vi "Robot Systems.vi"(11 "input cluster":T1) -> ()   [LabVIEW 2015]
uses:
  References/Refnums.vi
  Joystick/ControlsToCommands.ctl
panel:
  in  "Numeric":dbl
  out "YAxisLeft #2":dbl
  out "YAxisRight":dbl
  out "YAxisLeft":dbl
  out "XAxisLeft":dbl
  in  "Driving":u16(ring) items=["Manual", "Arcade", "Tank"]
  in  "Time Spinning before Index":dbl=5.0 caption="Delay Time (s)"
  in  "Time Indexing before Turning off Motors":dbl=3.0 caption="Delay Time (s)"
  in  "Motor Power":dbl min=-1.0 max=1.0 step=1.0
  in  "PWM 0":dbl min=-1.0 max=1.0
  in  "PWM 1":dbl min=-1.0 max=1.0
  in  "PWM 2":dbl min=-1.0 max=1.0
  in  "PWM 3":dbl min=-1.0 max=1.0
  in  "PWM 4":dbl min=-1.0 max=1.0
  in  "PWM 5":dbl min=-1.0 max=1.0
  in  "Apply Values":bool
  out "Boolean":bool
  in  "PWM 8":dbl min=-1.0 max=1.0 step=1.0
  # "THIS CANNOT BE ABORTED"
  # "MAYBE?"
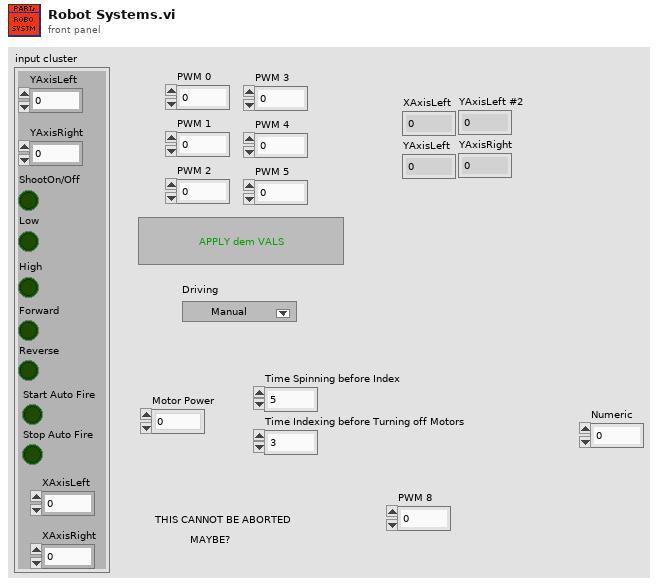
[diagram p1: front panel]
types:
  T1 = typedef "ControlsToCommands.ctl" = cluster{"YAxisLeft":dbl, "YAxisRight":dbl, "ShootOn/Off":bool, "Low":bool, "High":bool, "Forward":bool, "Reverse":bool, "Start Auto Fire":bool, "Stop Auto Fire":bool, "XAxisLeft":dbl, "XAxisRight":dbl}
  T2 = typedef "WPI_MotorControlDeviceRef.ctl" = cluster{"DeviceStatus":errorcluster, "Type":T3, "PWM":cluster{"PWM Channel":T4, "DeadBand":T5}, "CAN":cluster{"Device Number":u8, "Control Mode":T6, "Semaphore":T7, "Max Vout":dbl, "TalonSRX Control Mode":T8}, "Invert":bool}
  T3 = typedef "WPI_MotorControlType.ctl" = enum16{"PWM", "CAN", "CANTalonSRX"}
  T4 = typedef "FPGA_DIOPWMChannel.ctl" = enum8{"PWM 0", "PWM 1", "PWM 2", "PWM 3", "PWM 4", "PWM 5", "PWM 6", "PWM 7", "PWM 8", "PWM 9", "PWM MXP 0", "PWM MXP 1", "PWM MXP 2", "PWM MXP 3", "PWM MXP 4", "PWM MXP 5", "PWM MXP 6", "PWM MXP 7", "PWM MXP 8", "PWM MXP 9", "Invalid"}
  T5 = typedef "WPI_PWMDeadband.ctl" = cluster{"Name":string, "maxPositivePwm":i32, "minPositivePwm":i32, "centerPwm":i32, "maxNegativePwm":i32, "minNegativePwm":i32, "angularRange":u16}
  T6 = typedef "WPI_CANJaguar_ControlMode.ctl" = enum8{"Percent VBus", "Current", "Speed", "Position", "Voltage"}
  T7 = typedef "Semaphore RefNum" = refnum<k1>
  T8 = typedef "WPI_CANTalonSRX_APIControlMode.ctl" = enum8{"Percent VBus", "Speed", "Position", "Slave", "Unchanged / Invalid", "Voltage Compensation", "Current", "Motion Profile"}
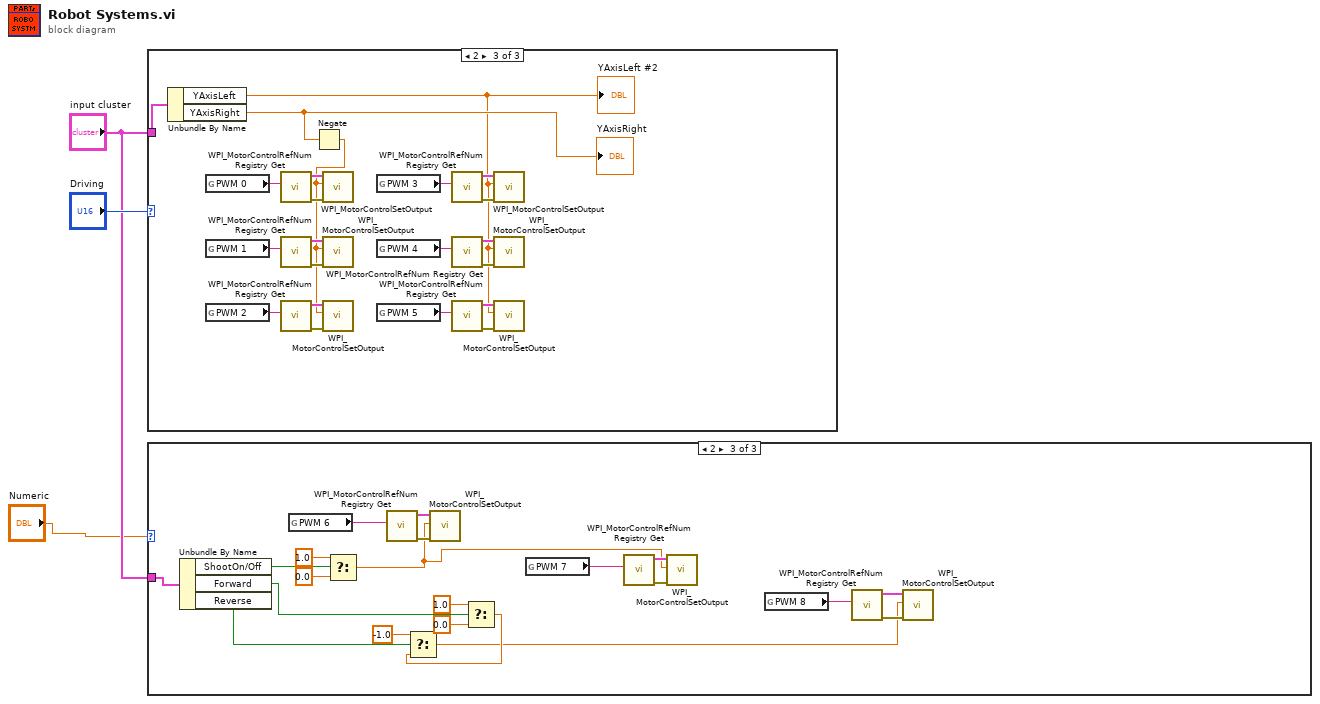
[diagram p0: block diagram]
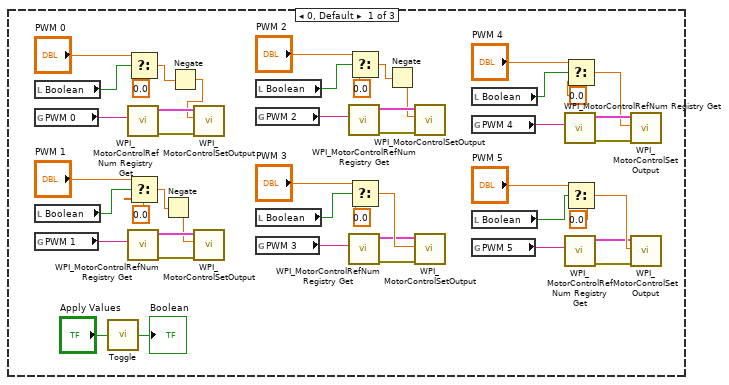
[diagram p2: hidden frame]
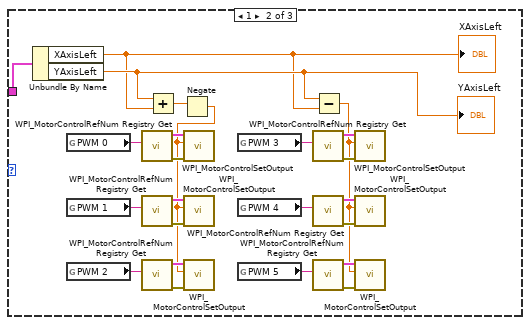
[diagram p3: hidden frame]
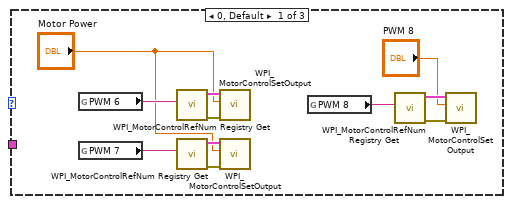
[diagram p4: hidden frame]
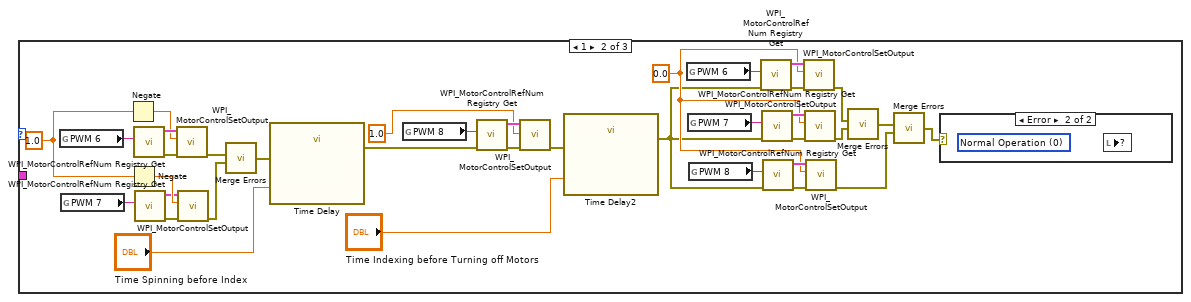
[diagram p5: hidden frame]
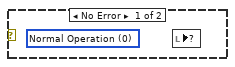
[diagram p6: hidden frame]
diagram:
  n1 = case shown="2" "Driving" {
    tunnel: "input cluster" -> [_ w74 w96]
    frame 0, Default {
      n2 = local read "Boolean"() -> (w34:bool)
      n3 = global read "Refnums.vi" "PWM 0"() -> (w23:string)
      n4 = local read "Boolean"() -> (w35:bool)
      n5 = global read "Refnums.vi" "PWM 1"() -> (w29:string)
      n6 = call "Toggle.vi"("Input"="Apply Values") -> ("Output"=→"Boolean":bool)  [unwired: 4 in]
      n7 = call <vilib>:"WPI_MotorControlRefNum Registry Get.vi"("refnum name"=w23) -> ("error out"=w25:errorcluster, "MotorControlDevRef"=w24:T2)  [unwired: 9 in]
      n8 = call <vilib>:"WPI_MotorControlRefNum Registry Get.vi"("refnum name"=w29) -> ("error out"=w31:errorcluster, "MotorControlDevRef"=w30:T2)  [unwired: 9 in]
      n9 = Select(t="PWM 0", s=w34, f=0.0) -> (s? t:f=w11:dbl)
      n10 = Select(t="PWM 1", s=w35, f=0.0) -> (s? t:f=w5:dbl)
      n11 = Negate(x=w5) -> (-x=w4:dbl)
      n12 = Negate(x=w11) -> (-x=w10:dbl)
      n13 = call <vilib>:"WPI_MotorControlSetOutput.vi"("error in (no error)"=w25, "Output"=w10, "MotorControlDevRef"=w24) -> ()  [unwired: 6 in, 3 out]
      n14 = call <vilib>:"WPI_MotorControlSetOutput.vi"("error in (no error)"=w31, "Output"=w4, "MotorControlDevRef"=w30) -> ()  [unwired: 6 in, 3 out]
      n15 = local read "Boolean"() -> (w37:bool)
      n16 = global read "Refnums.vi" "PWM 2"() -> (w28:string)
      n17 = local read "Boolean"() -> (w38:bool)
      n18 = global read "Refnums.vi" "PWM 3"() -> (w17:string)
      n19 = call <vilib>:"WPI_MotorControlRefNum Registry Get.vi"("refnum name"=w28) -> ("error out"=w26:errorcluster, "MotorControlDevRef"=w27:T2)  [unwired: 9 in]
      n20 = call <vilib>:"WPI_MotorControlRefNum Registry Get.vi"("refnum name"=w17) -> ("error out"=w19:errorcluster, "MotorControlDevRef"=w18:T2)  [unwired: 9 in]
      n21 = Select(t="PWM 2", s=w37, f=0.0) -> (s? t:f=w9:dbl)
      n22 = Select(t="PWM 3", s=w38, f=0.0) -> (s? t:f=w47:dbl)
      n23 = Negate(x=w9) -> (-x=w8:dbl)
      n24 = call <vilib>:"WPI_MotorControlSetOutput.vi"("error in (no error)"=w26, "Output"=w8, "MotorControlDevRef"=w27) -> ()  [unwired: 6 in, 3 out]
      n25 = call <vilib>:"WPI_MotorControlSetOutput.vi"("error in (no error)"=w19, "Output"=w47, "MotorControlDevRef"=w18) -> ()  [unwired: 6 in, 3 out]
      n26 = local read "Boolean"() -> (w41:bool)
      n27 = global read "Refnums.vi" "PWM 4"() -> (w16:string)
      n28 = local read "Boolean"() -> (w42:bool)
      n29 = global read "Refnums.vi" "PWM 5"() -> (w22:string)
      n30 = call <vilib>:"WPI_MotorControlRefNum Registry Get.vi"("refnum name"=w16) -> ("error out"=w14:errorcluster, "MotorControlDevRef"=w15:T2)  [unwired: 9 in]
      n31 = call <vilib>:"WPI_MotorControlRefNum Registry Get.vi"("refnum name"=w22) -> ("error out"=w20:errorcluster, "MotorControlDevRef"=w21:T2)  [unwired: 9 in]
      n32 = Select(t="PWM 4", s=w41, f=0.0) -> (s? t:f=w7:dbl)
      n33 = Select(t="PWM 5", s=w42, f=0.0) -> (s? t:f=w50:dbl)
      n34 = call <vilib>:"WPI_MotorControlSetOutput.vi"("error in (no error)"=w14, "Output"=w7, "MotorControlDevRef"=w15) -> ()  [unwired: 6 in, 3 out]
      n35 = call <vilib>:"WPI_MotorControlSetOutput.vi"("error in (no error)"=w20, "Output"=w50, "MotorControlDevRef"=w21) -> ()  [unwired: 6 in, 3 out]
    }
    frame 1 {
      n36 = Unbundle By Name(w74) -> ("XAxisLeft"=w54:dbl, "YAxisLeft"=w55:dbl)
      "XAxisLeft" <- w54
      "YAxisLeft" <- w55
      n37 = global read "Refnums.vi" "PWM 0"() -> (w70:string)
      n38 = global read "Refnums.vi" "PWM 1"() -> (w65:string)
      n39 = global read "Refnums.vi" "PWM 2"() -> (w58:string)
      n40 = call <vilib>:"WPI_MotorControlRefNum Registry Get.vi"("refnum name"=w70) -> ("error out"=w69:errorcluster, "MotorControlDevRef"=w68:T2)  [unwired: 9 in]
      n41 = call <vilib>:"WPI_MotorControlRefNum Registry Get.vi"("refnum name"=w65) -> ("error out"=w66:errorcluster, "MotorControlDevRef"=w67:T2)  [unwired: 9 in]
      n42 = call <vilib>:"WPI_MotorControlRefNum Registry Get.vi"("refnum name"=w58) -> ("error out"=w57:errorcluster, "MotorControlDevRef"=w56:T2)  [unwired: 9 in]
      n43 = Add(x=w55, y=w54) -> (x+y=w52:dbl)
      n44 = Negate(x=w52) -> (-x=w51:dbl)
      n45 = call <vilib>:"WPI_MotorControlSetOutput.vi"("error in (no error)"=w69, "Output"=w51, "MotorControlDevRef"=w68) -> ()  [unwired: 6 in, 3 out]
      n46 = call <vilib>:"WPI_MotorControlSetOutput.vi"("error in (no error)"=w66, "Output"=w51, "MotorControlDevRef"=w67) -> ()  [unwired: 6 in, 3 out]
      n47 = call <vilib>:"WPI_MotorControlSetOutput.vi"("error in (no error)"=w57, "Output"=w51, "MotorControlDevRef"=w56) -> ()  [unwired: 6 in, 3 out]
      n48 = global read "Refnums.vi" "PWM 3"() -> (w71:string)
      n49 = global read "Refnums.vi" "PWM 4"() -> (w64:string)
      n50 = global read "Refnums.vi" "PWM 5"() -> (w59:string)
      n51 = call <vilib>:"WPI_MotorControlRefNum Registry Get.vi"("refnum name"=w71) -> ("error out"=w73:errorcluster, "MotorControlDevRef"=w72:T2)  [unwired: 9 in]
      n52 = call <vilib>:"WPI_MotorControlRefNum Registry Get.vi"("refnum name"=w64) -> ("error out"=w62:errorcluster, "MotorControlDevRef"=w63:T2)  [unwired: 9 in]
      n53 = call <vilib>:"WPI_MotorControlRefNum Registry Get.vi"("refnum name"=w59) -> ("error out"=w61:errorcluster, "MotorControlDevRef"=w60:T2)  [unwired: 9 in]
      n54 = Subtract(x=w55, y=w54) -> (x-y=w53:dbl)
      n55 = call <vilib>:"WPI_MotorControlSetOutput.vi"("error in (no error)"=w73, "Output"=w53, "MotorControlDevRef"=w72) -> ()  [unwired: 6 in, 3 out]
      n56 = call <vilib>:"WPI_MotorControlSetOutput.vi"("error in (no error)"=w62, "Output"=w53, "MotorControlDevRef"=w63) -> ()  [unwired: 6 in, 3 out]
      n57 = call <vilib>:"WPI_MotorControlSetOutput.vi"("error in (no error)"=w61, "Output"=w53, "MotorControlDevRef"=w60) -> ()  [unwired: 6 in, 3 out]
    }
    frame 2 {
      n58 = Unbundle By Name(w96) -> ("YAxisLeft"=w75:dbl, "YAxisRight"=w76:dbl)
      "YAxisLeft #2" <- w75
      "YAxisRight" <- w76
      n59 = global read "Refnums.vi" "PWM 0"() -> (w92:string)
      n60 = global read "Refnums.vi" "PWM 1"() -> (w87:string)
      n61 = global read "Refnums.vi" "PWM 2"() -> (w80:string)
      n62 = call <vilib>:"WPI_MotorControlRefNum Registry Get.vi"("refnum name"=w92) -> ("error out"=w91:errorcluster, "MotorControlDevRef"=w90:T2)  [unwired: 9 in]
      n63 = call <vilib>:"WPI_MotorControlRefNum Registry Get.vi"("refnum name"=w87) -> ("error out"=w88:errorcluster, "MotorControlDevRef"=w89:T2)  [unwired: 9 in]
      n64 = call <vilib>:"WPI_MotorControlRefNum Registry Get.vi"("refnum name"=w80) -> ("error out"=w79:errorcluster, "MotorControlDevRef"=w78:T2)  [unwired: 9 in]
      n65 = Negate(x=w76) -> (-x=w77:dbl)
      n66 = call <vilib>:"WPI_MotorControlSetOutput.vi"("error in (no error)"=w91, "Output"=w77, "MotorControlDevRef"=w90) -> ()  [unwired: 6 in, 3 out]
      n67 = call <vilib>:"WPI_MotorControlSetOutput.vi"("error in (no error)"=w88, "Output"=w77, "MotorControlDevRef"=w89) -> ()  [unwired: 6 in, 3 out]
      n68 = call <vilib>:"WPI_MotorControlSetOutput.vi"("error in (no error)"=w79, "Output"=w77, "MotorControlDevRef"=w78) -> ()  [unwired: 6 in, 3 out]
      n69 = global read "Refnums.vi" "PWM 3"() -> (w93:string)
      n70 = global read "Refnums.vi" "PWM 4"() -> (w86:string)
      n71 = global read "Refnums.vi" "PWM 5"() -> (w81:string)
      n72 = call <vilib>:"WPI_MotorControlRefNum Registry Get.vi"("refnum name"=w93) -> ("error out"=w95:errorcluster, "MotorControlDevRef"=w94:T2)  [unwired: 9 in]
      n73 = call <vilib>:"WPI_MotorControlRefNum Registry Get.vi"("refnum name"=w86) -> ("error out"=w84:errorcluster, "MotorControlDevRef"=w85:T2)  [unwired: 9 in]
      n74 = call <vilib>:"WPI_MotorControlRefNum Registry Get.vi"("refnum name"=w81) -> ("error out"=w83:errorcluster, "MotorControlDevRef"=w82:T2)  [unwired: 9 in]
      n75 = call <vilib>:"WPI_MotorControlSetOutput.vi"("error in (no error)"=w95, "Output"=w75, "MotorControlDevRef"=w94) -> ()  [unwired: 6 in, 3 out]
      n76 = call <vilib>:"WPI_MotorControlSetOutput.vi"("error in (no error)"=w84, "Output"=w75, "MotorControlDevRef"=w85) -> ()  [unwired: 6 in, 3 out]
      n77 = call <vilib>:"WPI_MotorControlSetOutput.vi"("error in (no error)"=w83, "Output"=w75, "MotorControlDevRef"=w82) -> ()  [unwired: 6 in, 3 out]
    }
  }
  n78 = case shown="2" "Numeric" {
    tunnel: "input cluster" -> [_ _ w157]
    frame 0, Default {
      n79 = global read "Refnums.vi" "PWM 6"() -> (w105:string)
      n80 = global read "Refnums.vi" "PWM 7"() -> (w104:string)
      n81 = call <vilib>:"WPI_MotorControlRefNum Registry Get.vi"("refnum name"=w105) -> ("error out"=w106:errorcluster, "MotorControlDevRef"=w107:T2)  [unwired: 9 in]
      n82 = call <vilib>:"WPI_MotorControlRefNum Registry Get.vi"("refnum name"=w104) -> ("error out"=w102:errorcluster, "MotorControlDevRef"=w103:T2)  [unwired: 9 in]
      n83 = call <vilib>:"WPI_MotorControlSetOutput.vi"("error in (no error)"=w106, "Output"="Motor Power", "MotorControlDevRef"=w107) -> ()  [unwired: 6 in, 3 out]
      n84 = call <vilib>:"WPI_MotorControlSetOutput.vi"("error in (no error)"=w102, "Output"="Motor Power", "MotorControlDevRef"=w103) -> ()  [unwired: 6 in, 3 out]
      n85 = global read "Refnums.vi" "PWM 8"() -> (w100:string)
      n86 = call <vilib>:"WPI_MotorControlRefNum Registry Get.vi"("refnum name"=w100) -> ("error out"=w98:errorcluster, "MotorControlDevRef"=w99:T2)  [unwired: 9 in]
      n87 = call <vilib>:"WPI_MotorControlSetOutput.vi"("error in (no error)"=w98, "Output"="PWM 8", "MotorControlDevRef"=w99) -> ()  [unwired: 6 in, 3 out]
    }
    frame 1 {
      w116 = 0.0
      w135 = 1.0
      n88 = global read "Refnums.vi" "PWM 6"() -> (w140:string)
      n89 = global read "Refnums.vi" "PWM 7"() -> (w139:string)
      n90 = Negate(x=w135) -> (-x=w136:dbl)
      n91 = Negate(x=w135) -> (-x=w143:dbl)
      n92 = call <vilib>:"WPI_MotorControlRefNum Registry Get.vi"("refnum name"=w140) -> ("error out"=w141:errorcluster, "MotorControlDevRef"=w142:T2)  [unwired: 9 in]
      n93 = call <vilib>:"WPI_MotorControlRefNum Registry Get.vi"("refnum name"=w139) -> ("error out"=w137:errorcluster, "MotorControlDevRef"=w138:T2)  [unwired: 9 in]
      n94 = call <vilib>:"WPI_MotorControlSetOutput.vi"("error in (no error)"=w141, "Output"=w136, "MotorControlDevRef"=w142) -> ("error out"=w134:errorcluster)  [unwired: 6 in, 2 out]
      n95 = call <vilib>:"WPI_MotorControlSetOutput.vi"("error in (no error)"=w137, "Output"=w143, "MotorControlDevRef"=w138) -> ("error out"=w133:errorcluster)  [unwired: 6 in, 2 out]
      n96 = call "Merge Errors.vi"("error in 2"=w133, "error in"=w134) -> ("error out"=w132:errorcluster)  [unwired: 2 in]
      n97 = call "Time Delay"("error in (no error)"=w132, "Delay Time (s)"="Time Spinning before Index") -> ("error out"=w128:errorcluster)  [unwired: 9 in]
      n98 = global read "Refnums.vi" "PWM 8"() -> (w131:string)
      n99 = call <vilib>:"WPI_MotorControlRefNum Registry Get.vi"("error in (no error)"=w128, "refnum name"=w131) -> ("error out"=w130:errorcluster, "MotorControlDevRef"=w129:T2)  [unwired: 8 in]
      n100 = call <vilib>:"WPI_MotorControlSetOutput.vi"("error in (no error)"=w130, "Output"=1.0, "MotorControlDevRef"=w129) -> ("error out"=w126:errorcluster)  [unwired: 6 in, 2 out]
      n101 = call "Time Delay2"("error in (no error)"=w126, "Delay Time (s)"="Time Indexing before Turning off Motors") -> ("error out"=w115:errorcluster)  [unwired: 9 in]
      n102 = global read "Refnums.vi" "PWM 6"() -> (w122:string)
      n103 = global read "Refnums.vi" "PWM 7"() -> (w123:string)
      n104 = global read "Refnums.vi" "PWM 8"() -> (w119:string)
      n105 = call <vilib>:"WPI_MotorControlRefNum Registry Get.vi"("error in (no error)"=w115, "refnum name"=w122) -> ("error out"=w121:errorcluster, "MotorControlDevRef"=w120:T2)  [unwired: 8 in]
      n106 = call <vilib>:"WPI_MotorControlRefNum Registry Get.vi"("error in (no error)"=w115, "refnum name"=w123) -> ("error out"=w125:errorcluster, "MotorControlDevRef"=w124:T2)  [unwired: 8 in]
      n107 = call <vilib>:"WPI_MotorControlRefNum Registry Get.vi"("error in (no error)"=w115, "refnum name"=w119) -> ("error out"=w117:errorcluster, "MotorControlDevRef"=w118:T2)  [unwired: 8 in]
      n108 = call <vilib>:"WPI_MotorControlSetOutput.vi"("error in (no error)"=w121, "Output"=w116, "MotorControlDevRef"=w120) -> ("error out"=w110:errorcluster)  [unwired: 6 in, 2 out]
      n109 = call <vilib>:"WPI_MotorControlSetOutput.vi"("error in (no error)"=w125, "Output"=w116, "MotorControlDevRef"=w124) -> ("error out"=w109:errorcluster)  [unwired: 6 in, 2 out]
      n110 = call <vilib>:"WPI_MotorControlSetOutput.vi"("error in (no error)"=w117, "Output"=w116, "MotorControlDevRef"=w118) -> ("error out"=w111:errorcluster)  [unwired: 6 in, 2 out]
      n111 = call "Merge Errors.vi"("error in 2"=w109, "error in"=w110) -> ("error out"=w112:errorcluster)  [unwired: 2 in]
      n112 = call "Merge Errors.vi"("error in 2"=w111, "error in"=w112) -> ("error out"=w108:errorcluster)  [unwired: 2 in]
      n113 = case shown="Error" w108 {
        frame No Error {
          (unwired) u16 0 items=["Normal Operation", "Autonomous Shooting"] ("Shooting")
          n114 = local read item#-1() -> ()  [unwired: 1 in]
        }
        frame Error {
          (unwired) u16 0 items=["Normal Operation", "Autonomous Shooting"] ("Shooting")
          n115 = local read item#-1() -> ()  [unwired: 1 in]
        }
      }
    }
    frame 2 {
      n116 = Unbundle By Name(w157) -> ("ShootOn/Off"=w156:bool, "Forward"=w150:bool, "Reverse"=w149:bool)
      n117 = global read "Refnums.vi" "PWM 6"() -> (w161:string)
      n118 = Select(t=1.0, s=w156, f=0.0) -> (s? t:f=w152:dbl)
      n119 = call <vilib>:"WPI_MotorControlRefNum Registry Get.vi"("refnum name"=w161) -> ("error out"=w162:errorcluster, "MotorControlDevRef"=w153:T2)  [unwired: 9 in]
      n120 = call <vilib>:"WPI_MotorControlSetOutput.vi"("error in (no error)"=w162, "Output"=w152, "MotorControlDevRef"=w153) -> ()  [unwired: 6 in, 3 out]
      n121 = Select(t=1.0, s=w150, f=0.0) -> (s? t:f=w148:dbl)
      n122 = Select(t=-1.0, s=w149, f=w148) -> (s? t:f=w144:dbl)
      n123 = global read "Refnums.vi" "PWM 7"() -> (w160:string)
      n124 = call <vilib>:"WPI_MotorControlRefNum Registry Get.vi"("refnum name"=w160) -> ("error out"=w158:errorcluster, "MotorControlDevRef"=w159:T2)  [unwired: 9 in]
      n125 = call <vilib>:"WPI_MotorControlSetOutput.vi"("error in (no error)"=w158, "Output"=w152, "MotorControlDevRef"=w159) -> ()  [unwired: 6 in, 3 out]
      n126 = global read "Refnums.vi" "PWM 8"() -> (w164:string)
      n127 = call <vilib>:"WPI_MotorControlRefNum Registry Get.vi"("refnum name"=w164) -> ("error out"=w163:errorcluster, "MotorControlDevRef"=w151:T2)  [unwired: 9 in]
      n128 = call <vilib>:"WPI_MotorControlSetOutput.vi"("error in (no error)"=w163, "Output"=w144, "MotorControlDevRef"=w151) -> ()  [unwired: 6 in, 3 out]
    }
  }
